vi "Swerve Wheel.vi"(2 "Wheel":T1(ring)=enum."Front Right", 4 "Inputs":dbl[](array[numeric])=[0.0, 0.0, 0.0, 0.0, 0.0, 10.0, 14.727870051368596, 10.8125]) -> (0 "Speed":dbl, 1 "Angle":dbl)   [LabVIEW 2017]
panel:
  in  "RL Offset":dbl format="%#_13g"
  in  "RR Offset":dbl format="%#_13g"
  in  "FR Offset":dbl format="%#_13g"
  in  "FL Offset":dbl format="%#_13g"
  out "SetPoint":dbl
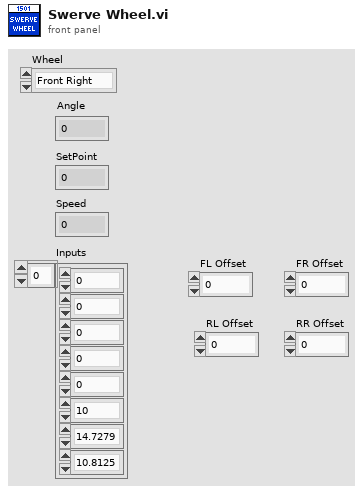
[diagram p1: front panel]
types:
  T1 = enum16{"Front Left", "Front Right", "Rear Right", "Rear Left"}
  T2 = enum16{"Z", "Y", "X", "Rot. Point X", "Rot. Point Y", "Width/2", "Max", "Length/2"}
  T3 = enum16{"Z Axis", "Y", "X", "Rot. Point X", "Rot. Point Y", "Width/2", "Max", "Length/2"}
  T4 = typedef "WPI_MotorControlDeviceRef.ctl" = cluster{"DeviceStatus":errorcluster, "Type":T5, "PWM":cluster{"PWM Channel":T6, "DeadBand":T7}, "CAN":cluster{"Device Number":u8, "SetOutput VI Ref":variant, "GetOutput VI Ref":variant, "Enable VI Ref":variant, "Disable VI Ref":variant, "Data":variant}, "Invert":bool, "DIO PWM":cluster{"PWM \"Enable\" Channel":T6, "DIOChannel":T8, "PWM Rate":dbl}}
  T5 = typedef "WPI_MotorControlType.ctl" = enum16{"PWM", "CAN", "DIO PWM"}
  T6 = typedef "FPGA_DIOPWMChannel.ctl" = enum8{"PWM 0", "PWM 1", "PWM 2", "PWM 3", "PWM 4", "PWM 5", "PWM 6", "PWM 7", "PWM 8", "PWM 9", "PWM MXP 0", "PWM MXP 1", "PWM MXP 2", "PWM MXP 3", "PWM MXP 4", "PWM MXP 5", "PWM MXP 6", "PWM MXP 7", "PWM MXP 8", "PWM MXP 9", "Invalid"}
  T7 = typedef "WPI_PWMDeadband.ctl" = cluster{"Name":string, "maxPositivePwm":i32, "minPositivePwm":i32, "centerPwm":i32, "maxNegativePwm":i32, "minNegativePwm":i32, "angularRange":u16}
  T8 = typedef "FPGA_DIOChannel.ctl" = enum8{"DIO 0", "DIO 1", "DIO 2", "DIO 3", "DIO 4", "DIO 5", "DIO 6", "DIO 7", "DIO 8", "DIO 9", "DIO MXP 0", "DIO MXP 1", "DIO MXP 2", "DIO MXP 3", "DIO MXP 4", "DIO MXP 5", "DIO MXP 6", "DIO MXP 7", "DIO MXP 8", "DIO MXP 9", "DIO MXP 10", "DIO MXP 11", "DIO MXP 12", "DIO MXP 13", "DIO MXP 14", "DIO MXP 15", "SPI Port CS1", "SPI Port CS2", "SPI Port CS3", "SPI Port MISO", "SPI Port MOSI", "Invalid"}
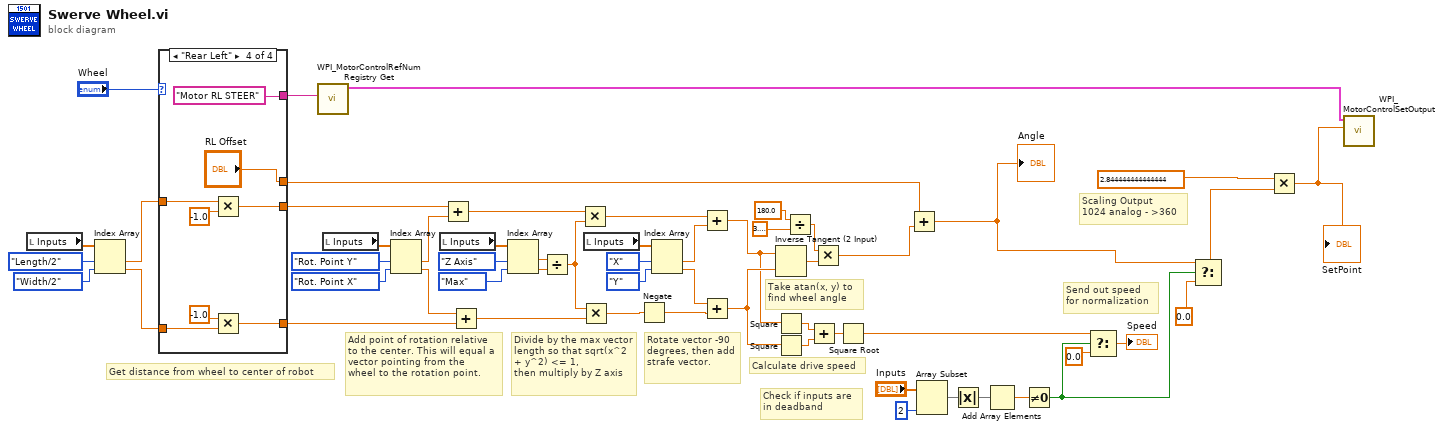
[diagram p0: block diagram]
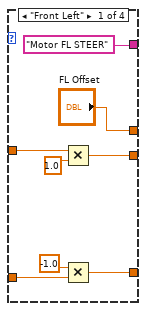
[diagram p2: hidden frame]
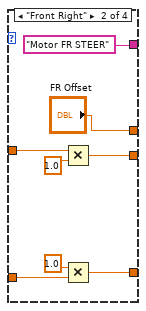
[diagram p3: hidden frame]
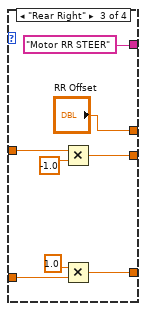
[diagram p4: hidden frame]
diagram:
  # "Scaling Output\n1024 analog - >360"
  # "Divide by the max vector length so that sqrt(x^2 + y^2) <= 1,\nthen multiply by Z axis"
  # "Add point of rotation relative to the center. This will equal a vector pointing from the\nwheel to the rotation point."
  # "Send out speed\nfor normalization"
  # "Check if inputs are\nin deadband"
  # "Take atan(x, y) to find wheel angle"
  # "Calculate drive speed"
  # "Rotate vector -90 degrees, then add strafe vector."
  # "Get distance from wheel to center of robot"
  n1 = local read "Inputs"() -> (w17:dbl[])
  n2 = Index Array(array=w17, index #1=T2."Length/2", index #2=T2."Width/2") -> (element #1=w15:dbl, element #2=w14:dbl)
  n3 = case shown="\"Rear Left\"" "Wheel" {
    tunnel: ["Motor FL STEER" "Motor FR STEER" "Motor RR STEER" "Motor RL STEER"] -> w11
    tunnel: ["FL Offset" "FR Offset" "RR Offset" "RL Offset"] -> w4
    tunnel: w15 -> [w62 w70 w78 w86]
    tunnel: w14 -> [w60 w68 w76 w84]
    tunnel: [w59 w67 w75 w83] -> w40
    tunnel: [w58 w66 w74 w82] -> w36
    frame "Front Left" {
      n4 = Multiply(x=w62, y=1.0) -> (x*y=w59:dbl)
      n5 = Multiply(x=-1.0 ("y"), y=w60) -> (x*y=w58:dbl)
    }
    frame "Front Right" {
      n6 = Multiply(x=w70, y=1.0) -> (x*y=w67:dbl)
      n7 = Multiply(x=1.0 ("y"), y=w68) -> (x*y=w66:dbl)
    }
    frame "Rear Right" {
      n8 = Multiply(x=w78, y=-1.0) -> (x*y=w75:dbl)
      n9 = Multiply(x=1.0 ("y"), y=w76) -> (x*y=w74:dbl)
    }
    frame "Rear Left" {
      n10 = Multiply(x=w86, y=-1.0) -> (x*y=w83:dbl)
      n11 = Multiply(x=-1.0 ("y"), y=w84) -> (x*y=w82:dbl)
    }
  }
  n12 = call <vilib>:"WPI_MotorControlRefNum Registry Get.vi"("refnum name"=w11) -> ("MotorControlDevRef"=w3:T4)  [unwired: 9 in, 1 out]
  n13 = local read "Inputs"() -> (w38:dbl[])
  n14 = Index Array(array=w38, index #1=T2."Rot. Point Y", index #2=T2."Rot. Point X") -> (element #1=w34:dbl, element #2=w35:dbl)
  n15 = local read "Inputs"() -> (w32:dbl[])
  n16 = Add(x=w40, y=w34) -> (x+y=w12:dbl)
  n17 = Add(x=w35, y=w36) -> (x+y=w28:dbl)
  n18 = Index Array(array=w32, index #1=T3."Z Axis", index #2=T2."Max") -> (element #1=w29:dbl, element #2=w30:dbl)
  n19 = Divide(x=w29, y=w30) -> (x/y=w27:dbl)
  n20 = Multiply(x=w12, y=w27) -> (x*y=w13:dbl)
  n21 = Multiply(x=w27, y=w28) -> (x*y=w2:dbl)
  n22 = local read "Inputs"() -> (w25:dbl[])
  n23 = Negate(x=w2) -> (-x=w1:dbl)
  n24 = Index Array(array=w25, index #1=T2."X", index #2=T2."Y") -> (element #1=w21:dbl, element #2=w22:dbl)
  n25 = Add(x=w13, y=w21) -> (x+y=w19:dbl)
  n26 = Add(x=w22, y=w1) -> (x+y=w20:dbl)
  n27 = Inverse Tangent (2 Input)(1:w20, 2:w19) -> (0:w53:dbl)
  n28 = Square(x=w19) -> (x^2=w23:dbl)
  n29 = Square(x=w20) -> (x^2=w52:dbl)
  n30 = Divide(x=180.0 ("y"), y=3.141592653589793) -> (x/y=w50:dbl)
  n31 = Add(x=w23, y=w52) -> (x+y=w51:dbl)
  n32 = Multiply(x=w50, y=w53) -> (x*y=w6:dbl)
  n33 = Square Root(x=w51) -> (sqrt(x)=w7:dbl)
  n34 = Add(x=w4, y=w6) -> (x+y=w5:dbl)
  "Angle" <- w5
  n35 = Array Subset(array="Inputs", length=2) -> (w45:dbl[])  [unwired: 1 in]
  n36 = Absolute Value(x=w45) -> (abs(x)=w41:dbl[])
  n37 = Add Array Elements(numeric array=w41) -> (sum=w54:dbl)
  n38 = Not Equal To 0?(x=w54) -> (x != 0?=w42:bool)
  n39 = Select(t=w7, s=w42, f=0.0) -> (s? t:f=→"Speed":dbl)
  n40 = Select(t=w5, s=w42, f=0.0) -> (s? t:f=w10:dbl)
  n41 = Multiply(x=2.844444444444444 ("y"), y=w10) -> (x*y=w9:dbl)
  "SetPoint" <- w9
  n42 = call <vilib>:"WPI_MotorControlSetOutput.vi"("Output"=w9, "MotorControlDevRef"=w3) -> ()  [unwired: 7 in, 3 out]
